vi "Test UDP Command Receive.vi"(8 "Target port":u16=8889, 9 "receiver port":u16=8888, 10 "Test Input":string="testcommand", 11 "VeriStand Target address":string="127.0.0.1") -> (0 "error out":errorcluster, 3 "Command Receivd?":bool)   [LabVIEW 2015]
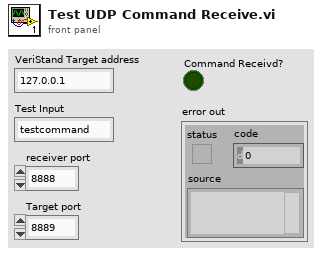
[diagram p1: front panel]
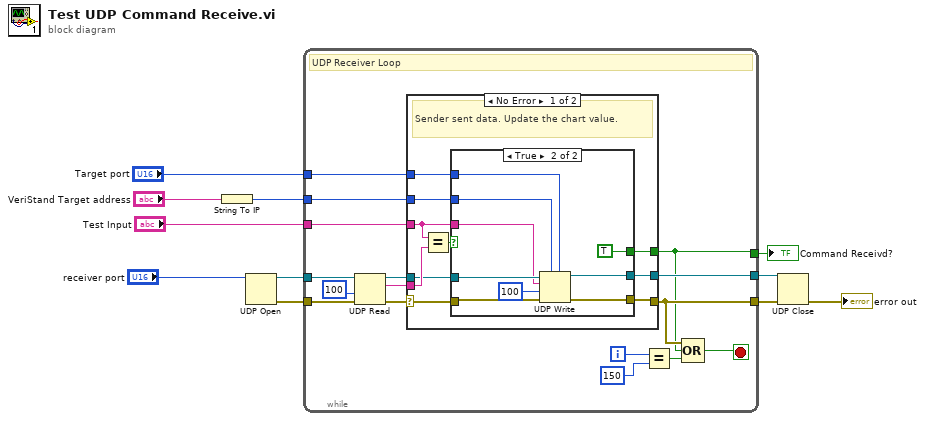
[diagram p0: block diagram]
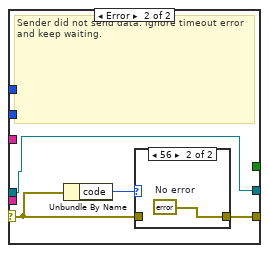
[diagram p3: hidden frame]
diagram:
  n1 = String To IP(1:"VeriStand Target address") -> (0:w6:u32)
  n2 = UDP Open(11:"receiver port") -> (port=w3:refnum<k16>, 0:w2:errorcluster)  [unwired: 4 in, 1 out]
  n3 = while {
    tunnel: w3 -> [w27]
    tunnel: w2 -> [w26]
    tunnel: [w17] -> w1
    tunnel: "Test Input" -> [w22]
    tunnel: w6 -> [w20]
    tunnel: "Target port" -> [w19]
    tunnel: [w18] -> w9
    tunnel: [w15] -> w10
    i -> [w14]
    stop <- w16 stop-if-true
    # "UDP Receiver Loop"
    n4 = UDP Read(connection ID=w27, timeout ms (25000)=100, 8:w26) -> (data out=w24:string, error out=w23:errorcluster, 3:w21:refnum<k16>)  [unwired: 3 out]
    n5 = case shown="No Error" w23 {
      selector: w23 -> [w36 w51]
      tunnel: w24 -> [w37 _]
      tunnel: [w33 w50] -> w17
      tunnel: w22 -> [w32 _]
      tunnel: w21 -> [w34 w49]
      tunnel: w20 -> [w31 _]
      tunnel: w19 -> [w30 _]
      tunnel: [w29 w49] -> w18
      tunnel: [w28 _] -> w15
      frame No Error {
        # "Sender sent data. Update the chart value."
        n6 = Equal?(x=w32, y=w37) -> (x = y?=w35:bool)
        n7 = case shown="True" w35 {
          tunnel: w36 -> [w38 w47]
          tunnel: w34 -> [w39 w48]
          tunnel: [w38 w46] -> w33
          tunnel: w32 -> [_ w45]
          tunnel: w31 -> [_ w43]
          tunnel: w30 -> [_ w42]
          tunnel: [w39 w41] -> w29
          tunnel: [_ TRUE] -> w28
          frame False {
          }
          frame True {
            n8 = UDP Write(address=w43, port or service name=w42, connection ID=w48, data in=w45, 8:w47, 9:100 ("timeout ms (25000)")) -> (error out=w46:errorcluster, 3:w41:refnum<k16>)
          }
        }
      }
      frame Error {
        # "Sender did not send data. Ignore timeout error and keep waiting."
        n9 = Unbundle By Name(w51) -> ("code"=w52:i32)
        n10 = case shown="56" w52 {
          tunnel: w51 -> [w53 _]
          tunnel: [w53 w54] -> w50
          frame Default {
          }
          frame 56 {
            w54 = errorcluster {"status"=FALSE, "code"=0, "source"=""}  # No error
          }
        }
      }
    }
    n11 = Equal?(x=w14, y=150) -> (x = y?=w12:bool)
    n12 = Compound Arithmetic op=OR(w17, w15, w12) -> (w16:bool)
  }
  "Command Receivd?" <- w10
  n13 = UDP Close(connection ID=w9, 8:w1) -> (error out=→"error out":errorcluster)  [unwired: 1 out]
